vi "test_BuildEvalStr_Boolean-pos.vi"(8 "error in (no error)":errorcluster, 11 "TestCase in":refnum<class "Build Eval Str Test Case.lvclass">) -> (0 "error out":errorcluster, 3 "TestCase out":refnum<class "Build Eval Str Test Case.lvclass">)   [LabVIEW 2018, in "Build Eval Str Test Case.lvclass"]
uses:
  Build Eval Str Test Case.lvclass
  Plugins/Utility/Test Classes/Boolean/Boolean.lvclass
  C:/Users/UKHornP/Documents/Work/Projects/Assert API/Plugins/Utility/Test Classes/Test.lvclass
  Plugins/Utility/Test Classes/Test Class String IDs.vi
  <vilib>/addons/_JKI Toolkits/VI Tester/TestCase.llb/TestCase.lvclass
  Plugins/Utility/Test Classes/Test.lvclass
  C:/Program Files (x86)/National Instruments/LabVIEW 2018/vi.lib/addons/_JKI Toolkits/VI Tester/TestCase.llb/TestCase.lvclass
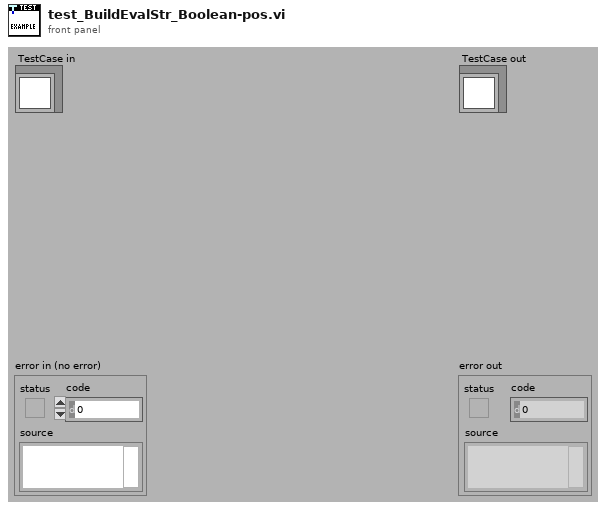
[diagram p1: front panel]
types:
  T1 = cluster{"Comparison Value 1":string, "Comparison Value 2":string, "Invert Result":string, "Assert VI Name":string, "Data Type":string, "Builder User Name":string, "Build Timestamp":string, "Failure Action":string, "Comment":string, "Assert Name":string, "Description":string, "Evaluation String":string}
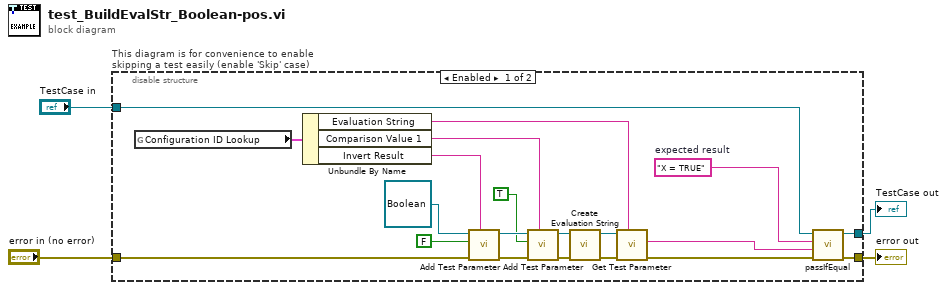
[diagram p0: block diagram]
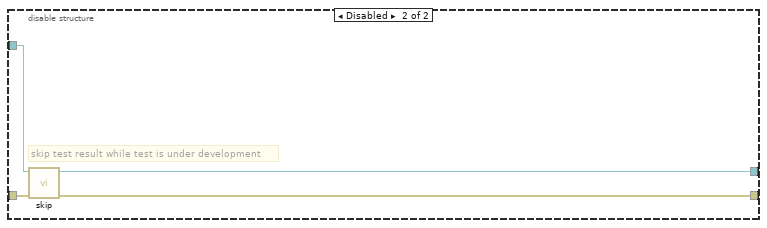
[diagram p2: hidden frame]
diagram:
  n1 = disable-structure "This diagram is for convenience to enable skipping a test easily (enable 'Skip' case)" shown="Enabled" {
    disable-tunnel: "TestCase in" -> [w23 w28]
    disable-tunnel: [w22 w26] -> w1
    disable-tunnel: [w21 w27] -> w3
    disable-tunnel: "error in (no error)" -> [w13 w25]
    frame Enabled {
      w24 = "X = TRUE"  # expected result
      n2 = global read "Test Class String IDs.vi" "Configuration ID Lookup"() -> (w19:T1)
      n3 = Unbundle By Name(w19) -> ("Evaluation String"=w6:string, "Comparison Value 1"=w17:string, "Invert Result"=w18:string)
      n4 = call-dynamic "Add Test Parameter.vi"("Data Value ID"=w18, "error in (no error)"=w13, "Data Value"=FALSE, "Test in"=refnum<class "Boolean.lvclass"> refnum ("Boolean.lvclass")) -> ("error out"=w12:errorcluster, "Test out"=w16:refnum<class "Boolean.lvclass">)  [unwired: 5 in, 1 out]
      n5 = call-dynamic "Add Test Parameter.vi"("Data Value ID"=w17, "error in (no error)"=w12, "Data Value"=TRUE, "Test in"=w16) -> ("error out"=w10:errorcluster, "Test out"=w11:refnum<class "Boolean.lvclass">)  [unwired: 5 in, 1 out]
      n6 = call-dynamic "Create Evaluation String.vi"("error in (no error)"=w10, "Boolean in"=w11) -> ("error out"=w9:errorcluster, "Boolean out"=w7:refnum<class "Boolean.lvclass">)  [unwired: 8 in]
      n7 = call "Get Test Parameter.vi"("Data Value ID"=w6, "error in (no error)"=w9, "Test in"=w7) -> ("error out"=w8:errorcluster, "Test Parameter"=w5:string)  [unwired: 6 in, 1 out]
      n8 = call-dynamic "passIfEqual.vi"("error in (no error)"=w8, "y"=w5, "x"=w24, "TestCase in"=w23) -> ("error out"=w21:errorcluster, "TestCase out"=w22:refnum<class "Build Eval Str Test Case.lvclass">)  [unwired: 6 in]
    }
    frame Disabled {
      # "skip test result while test is under development"
      n9 = call <vilib>:"skip.vi"("error in (no error)"=w25, "TestCase in"=w28) -> ("error out"=w27:errorcluster, "TestCase out"=w26:refnum<class "Build Eval Str Test Case.lvclass">)  [unwired: 8 in]
    }
  }
  "error out" <- w3
  "TestCase out" <- w1
